vi "Open.vi"   [LabVIEW 2021, in "Field_RnD_Services_LIBSSH2_Toolkit.lvlib" / "SFTP File.lvclass"]
doc: "Creates a new SFTP File object that represents a libssh2lv shared library SFTP File struct. This VI must be called, or executed, before using any other SFTP File-related VIs. This VI allocates memory within the libssh2lv shared library that must be explicitly deallocated, or freed, at the end of the application using the <B>Close</B> VI to avoid memory leaks or running Out-of-Memory (OOM) on a resource contrained system.\n\nA SFTP File object represents an existing file on a remote SFTP filesystem."
uses:
  220524-VNA RP FLAT.llb/SFTP File.lvclass
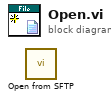
[diagram p0: block diagram]
diagram:
  n1 = call "Open from SFTP.vi"() -> ()  [unwired: 10 in, 2 out]
